vi "Batch Start.vi"(8 "error in":errorcluster, 10 "Test Result In":T2, 11 "CalCfg File In":T1) -> (0 "error out":errorcluster, 1 "Pass":bool, 2 "Test Result Out":T2, 3 "CalCfg File Out":T1, 4 "String":string)   [LabVIEW 2020, in "GUCalibration2.lvlib"]
uses:
  GUCalibration2.lvlib
  Controls/Test Result.ctl
  Controls/Site Data Element.ctl
  Controls/Site Raw Data Element.ctl
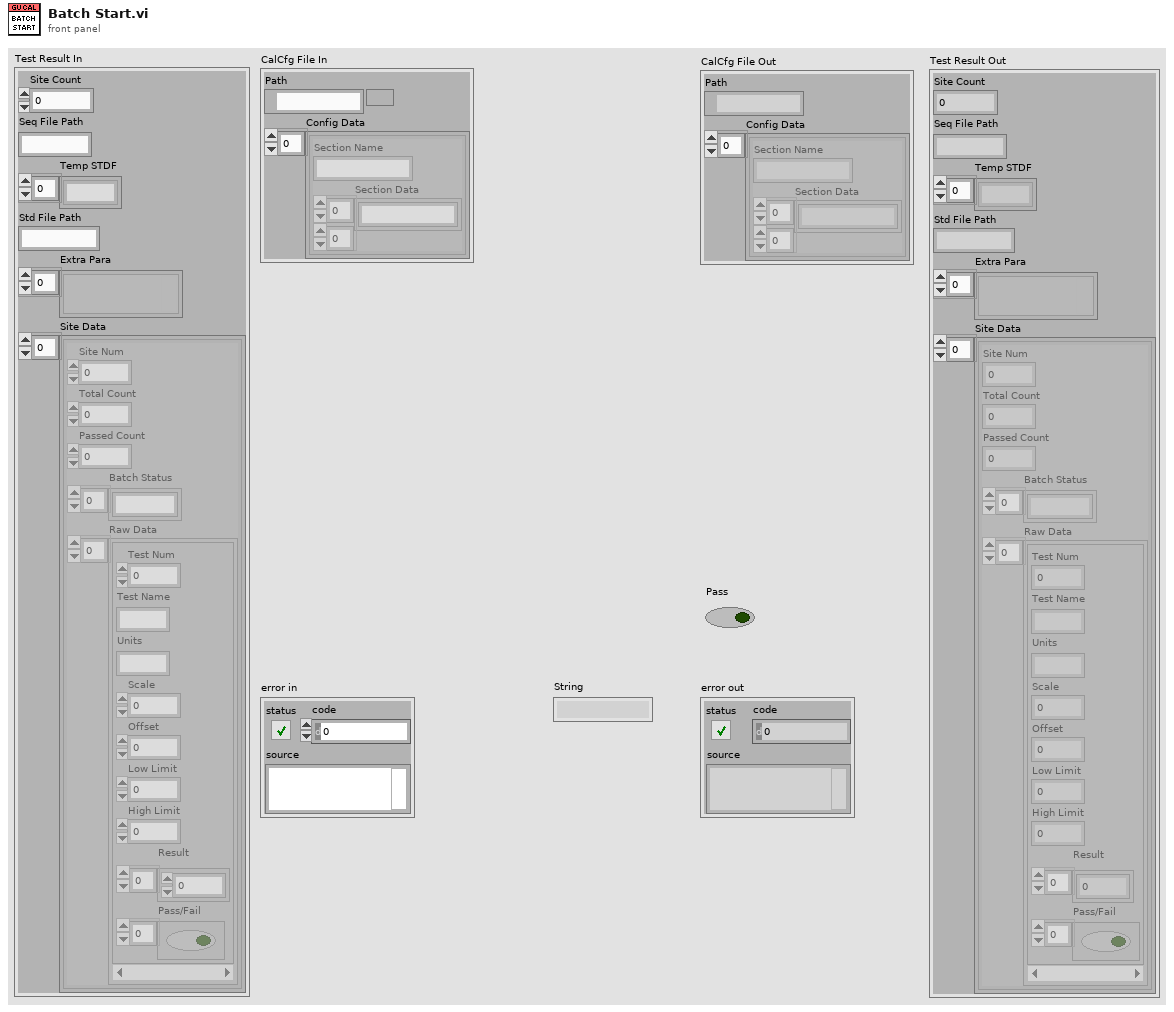
[diagram p1: front panel]
types:
  T1 = cluster{"Path":path, "Config Data":cluster{"Section Name":string, "Section Data":string[][]}[]}
  T2 = typedef "GUCalibration2.lvlib/Test Result.ctl" = cluster{"Site Count":i32, "Seq File Path":string, "Temp STDF":string[], "Std File Path":string, "Extra Para":variant[], "Site Data":T3[]}
  T3 = typedef "GUCalibration2.lvlib/Site Data Element.ctl" = cluster{"Site Num":i32, "Total Count":i32, "Passed Count":i32, "Batch Status":string[], "Raw Data":T4[]}
  T4 = typedef "GUCalibration2.lvlib/Site Raw Data Element.ctl" = cluster{"Test Num":u32, "Test Name":string, "Units":string, "Scale":i8, "Offset":dbl, "Low Limit":dbl, "High Limit":dbl, "Result":dbl[], "Pass/Fail":bool[]}
  T5 = cluster{"Section Name":string, "Section Data":string[][]}[]
  T6 = typedef "GUCalibration2.lvlib/Config Data Type.ctl" = cluster{"Cal Type":i32, "Curr Batch Index":i32, "Loop Count Per GU":i32, "Min Num of Pass GUs Per Site":i32, "Is Calibration":bool, "Batch Iteration Done":bool, "Cal Abort":bool, "Update Offset":bool, "Cal Check Pass":bool, "Cal End":bool, "Enabled Site":i32[], "GU Selected":i32[], "All Available GU":i32[], "GU Arrange":i32[][], "Batch Test Count":i32[][], "Batch Test Result":string[][], "Curr Batch":i32[], "Curr Batch Test Count":i32[], "Curr Batch Target Count":i32[], "Curr Batch Test Result":string[]}
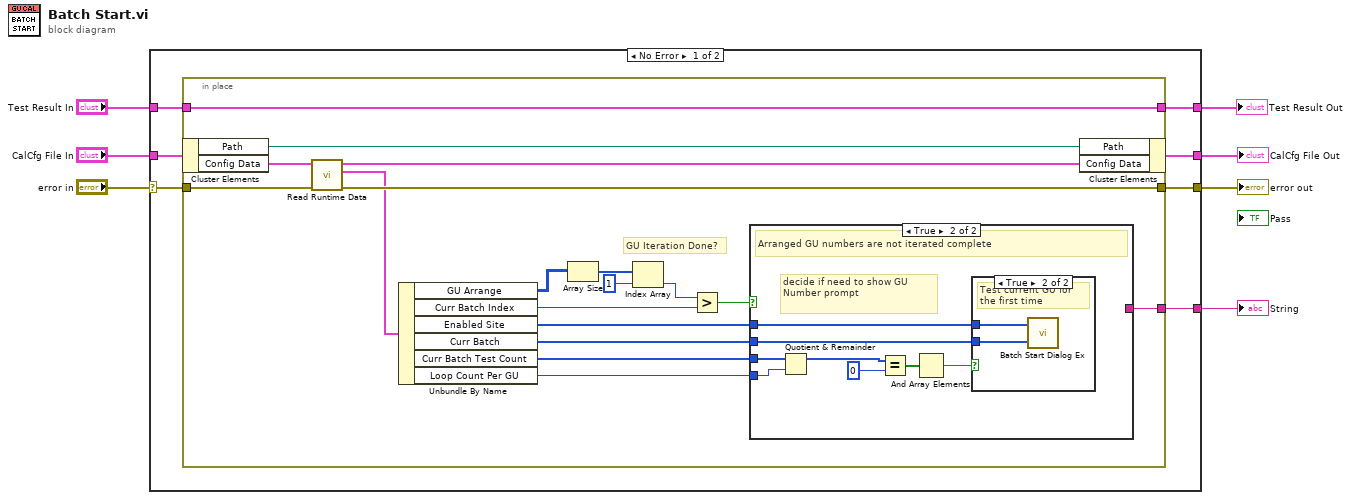
[diagram p0: block diagram]
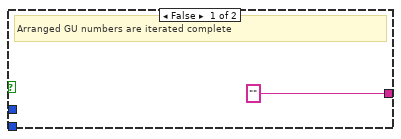
[diagram p2: hidden frame]
diagram:
  n1 = case shown="No Error" "error in" {
    selector: "error in" -> [w12 w46]
    tunnel: "Test Result In" -> [w14 w44]
    tunnel: "CalCfg File In" -> [w11 w45]
    tunnel: [w13 w46] -> w5
    tunnel: [w10 w45] -> w3
    tunnel: [w9 w44] -> w2
    tunnel: [w8 _] -> w1
    frame No Error {
      n2 = in-place {
        in-place-border: w14 -> [w17]
        in-place-border: [w31] -> w13
        in-place-border: w12 -> [w32]
        in-place-border: [w17] -> w9
        in-place-border: [w16] -> w8
        # "GU Iteration Done?"
        n3 = in-place-cluster #1(w11) -> ("Path"=w28:path, "Config Data"=w29:T5)
        n4 = call "Read Runtime Data.vi"("error in"=w32, "Config File Data In"=w29) -> ("error out"=w31:errorcluster, "Runtime Data Out"=w24:T6, "Config Data Out"=w30:T5)  [unwired: 7 in]
        n5 = Unbundle By Name(w24) -> ("GU Arrange"=w21:i32[][], "Curr Batch Index"=w19:i32, "Enabled Site"=w26:i32[], "Curr Batch"=w27:i32[], "Curr Batch Test Count"=w25:i32[], "Loop Count Per GU"=w15:i32)
        n6 = Array Size(array=w21) -> (size(s)=w23:i32[])
        n7 = Index Array(array=w23, index=1) -> (element=w20:i32)
        n8 = Greater?(x=w20, y=w19) -> (0:w18:bool)
        n9 = case shown="True" w18 {
          tunnel: w27 -> [_ w41]
          tunnel: w26 -> [_ w40]
          tunnel: w25 -> [_ w37]
          tunnel: ["" ("String") _] -> w16
          tunnel: w15 -> [_ w36]
          frame False {
            # "Arranged GU numbers are iterated complete"
          }
          frame True {
            # "decide if need to show GU Number prompt"
            # "Arranged GU numbers are not iterated complete"
            n10 = Quotient & Remainder(x=w37, y=w36) -> (x-y*floor(x/y)=w35:i32[])  [unwired: 1 out]
            n11 = Equal?(x=w35, y=0) -> (x = y?=w38:bool[])
            n12 = And Array Elements(Boolean array=w38) -> (logical AND=w39:bool)
            n13 = case shown="True" w39 {
              tunnel: w40 -> [_ w43]
              tunnel: w41 -> [_ w42]
              frame False {
              }
              frame True {
                # "Test current GU for the first time"
                n14 = call "Batch Start Dialog Ex.vi"("Curr GU"=w42, "Enabled Site"=w43) -> ()  [unwired: 1 out]
              }
            }
          }
        }
        n15 = in-place-cluster #1("Path"=w28, "Config Data"=w30) -> (w10:T1)
      }
    }
    frame Error {
    }
  }
  "error out" <- w5
  "CalCfg File Out" <- w3
  "Test Result Out" <- w2
  "String" <- w1
